vi "humidity_sensing_v_1.vi"() -> ()   [LabVIEW 2014]
doc: "This example shows how to configure a measurement and take a reading."
uses:
  <instrlib>/Keithley 24XX/Public/Data/Read (Single Point).vi
  <instrlib>/Keithley 24XX/Keithley 24XX.lvlib
panel:
  out "xxxxx":string
  in  "xxxxx":path=path "C:/Users/Administrator/Documents/Device-characterization-setup/IV-Trace/Data/dumb/2015_xx_xx_xxxx_xx_keithley_resistivity_001.txt"
  out "xxx":cluster{sgl[], i32[]}(graph)
  out "Data Real Time  Current":string
  in  "Data Real Time Current":path=path "C:/Users/Administrator/Documents/Device-characterization-setup/IV-Trace/Data/dumb/2015_xx_xx_xxxx_xx_keithley_resistivity_001.txt"
  out "Current-Sample Number":cluster{sgl[], i32[]}(graph)
  out "Analog Data 4":sgl(graph)
  out "Analog Data 3":sgl(graph)
  in  "loop num":dbl=1.0
  out "Data Resistivity":string
  in  "Data Resistivity":path=path "C:/Users/Administrator/Documents/Device-characterization-setup/IV-Trace/Data/dumb/2015_xx_xx_xxxx_xx_keithley_resistivity_001.txt"
  out "Resistance-Voltage":cluster{sgl[], sgl[]}(graph)
  in  "current multiplier":dbl=1.0
  out "Data IV Keithley":string
  in  "Data IV Keithley":path=path "C:/Users/Administrator/Documents/Device-characterization-setup/IV-Trace/Data/dumb/2015_xx_xx_xxxx_xx_keithley_001.txt"
  out "IV Curve":cluster{sgl[], dbl[]}(graph)
  in  "Stop Voltage/Current":dbl=2.0
  in  "Step":dbl=1.0
  in  "Source Mode  (0: Voltage)":u16(ring) items=["Voltage", "Current"]
  in  "Compliance  Level (0.1)":dbl=1.0
  in  "Start Voltage/Current":dbl
  in  "Enable Resistance Auto Range (T:Enable)":bool
  in  "Enable Current Auto Range (T:Enable)":bool=TRUE
  in  "Enable Voltage Auto Range (T:Enable)":bool
  in  "Resistance Manual Range (1.0)":dbl=1.0
  in  "Current Manual Range (1.0)":dbl=1.0
  in  "Voltage Manual Range (1.0)":dbl=1.0
  out "Resistance":sgl
  out "Current":sgl
  out "Voltage":sgl
  in  "Serial Configuration":T1={"Baud Rate"=9600, "Parity"=0, "Data Bits"=8, "Stop Bits"=10, "Flow Control"=0} {"Flow Control" items=["None", "XON/XOFF", "RTS/CTS", "XON/XOFF & RTS/CTS", "DTR/DSR", "XON/XOFF & DTR/DSR"]; "Stop Bits" items=["1.0"=10, "1.5"=15, "2.0"=20]; "Data Bits" items=["7"=7, "8"=8]; "Parity" items=["None", "Odd", "Even", "Mark", "Space"]; "Baud Rate" items=["300"=300, "600"=600, "1200"=1200, "2400"=2400, "4800"=4800, "9600"=9600, "19200"=19200]}
  in  "VISA resource name":refnum<visa-resource-name>="GPIB9::24::INSTR"
  # "NanoBEEs 2015-IV Tracer v1.0"
  # "Source Settings"
  # "GPIB9::24::INSTR"
  # "Voltage Range Settings"
  # "Current Range Settings"
  # "This multiplies the current value\nwith the number that entered, in order\nto  graph lower current values."
  # "Resistance Range Settings"
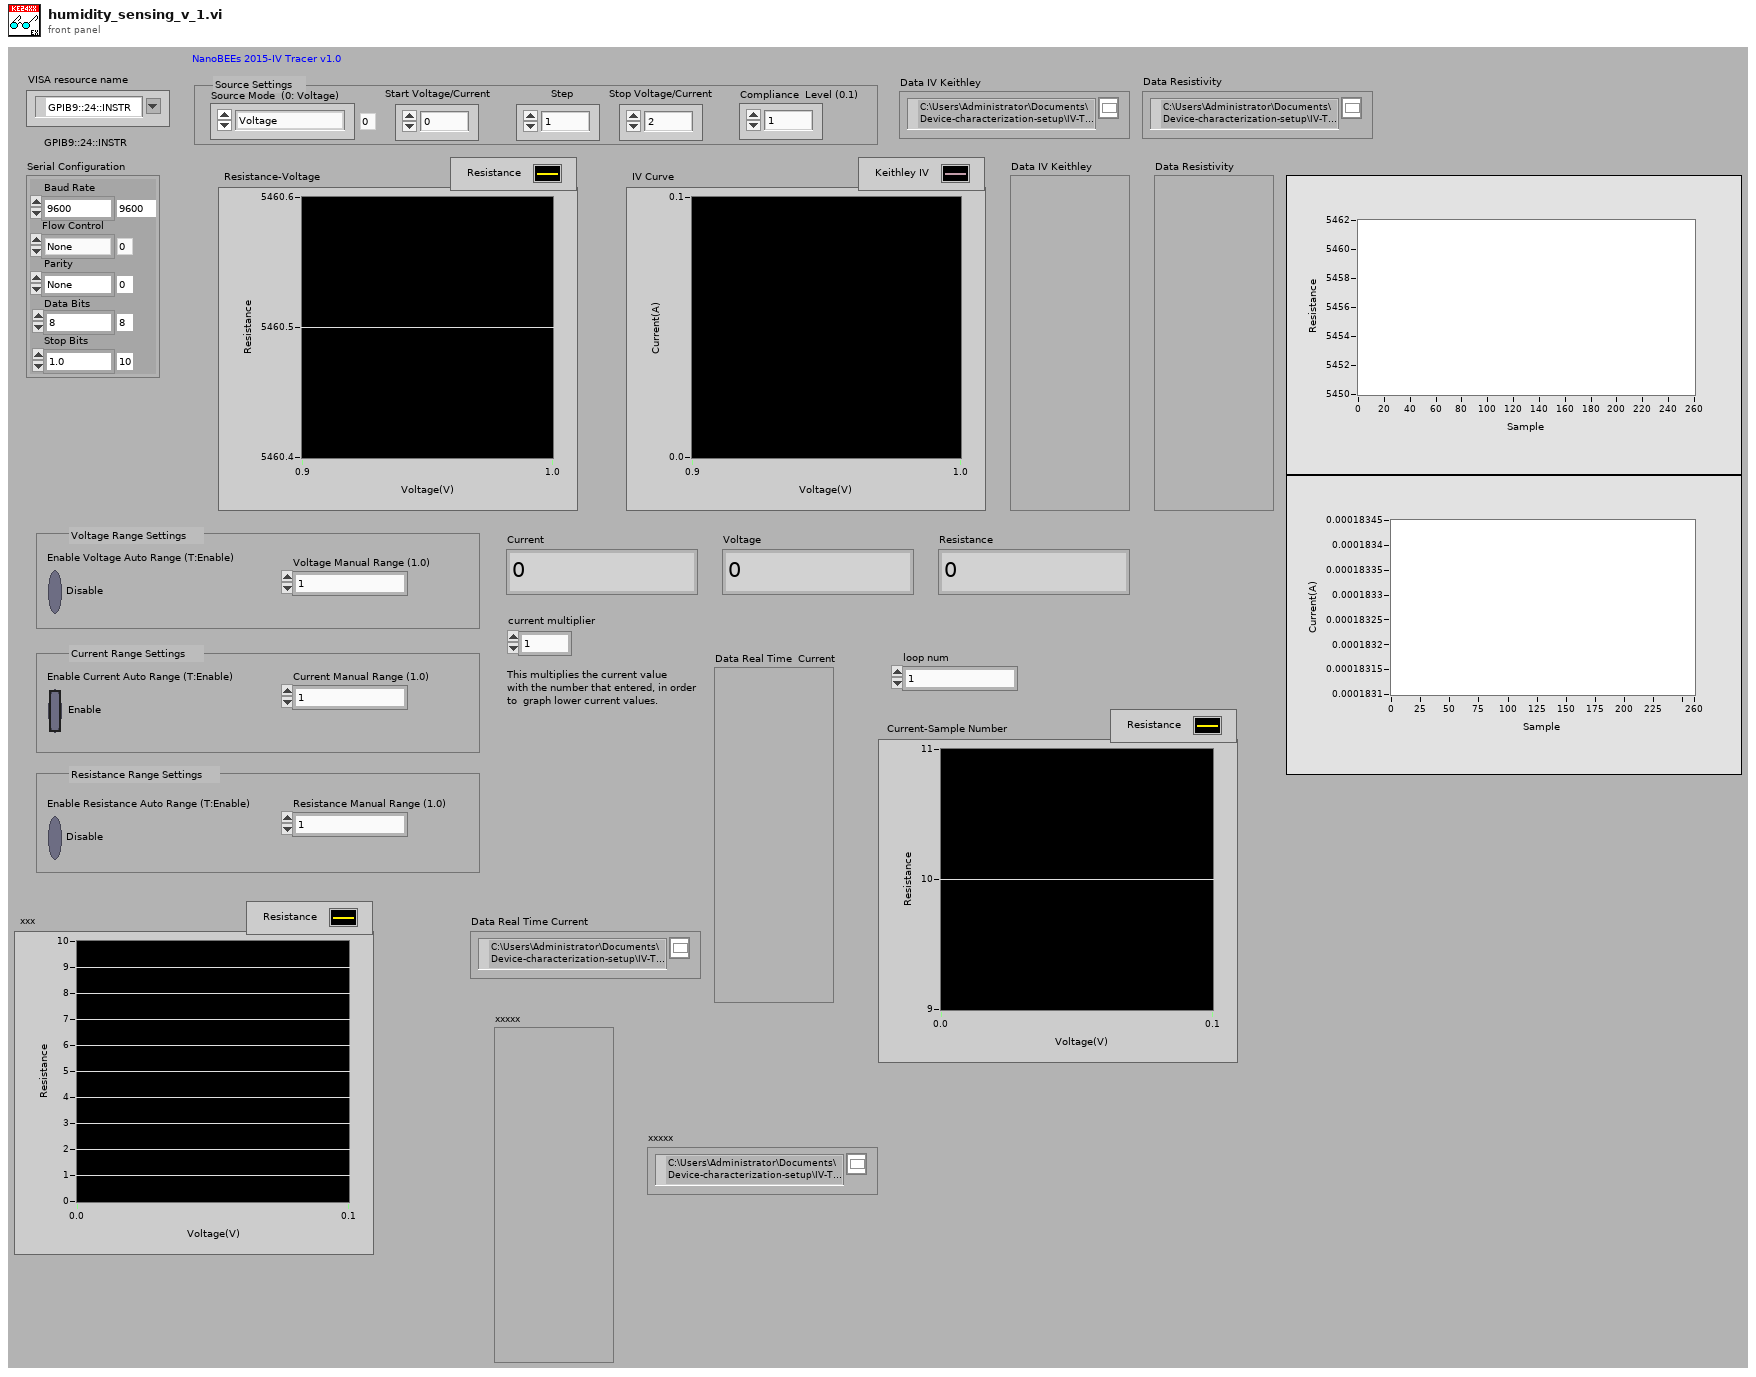
[diagram p1: front panel]
types:
  T1 = cluster{"Baud Rate":u32, "Parity":u16, "Data Bits":u16, "Stop Bits":u16, "Flow Control":u16}
  T2 = enum16{"open", "replace", "create", "open or create", "replace or create", "replace or create with confirmation"}
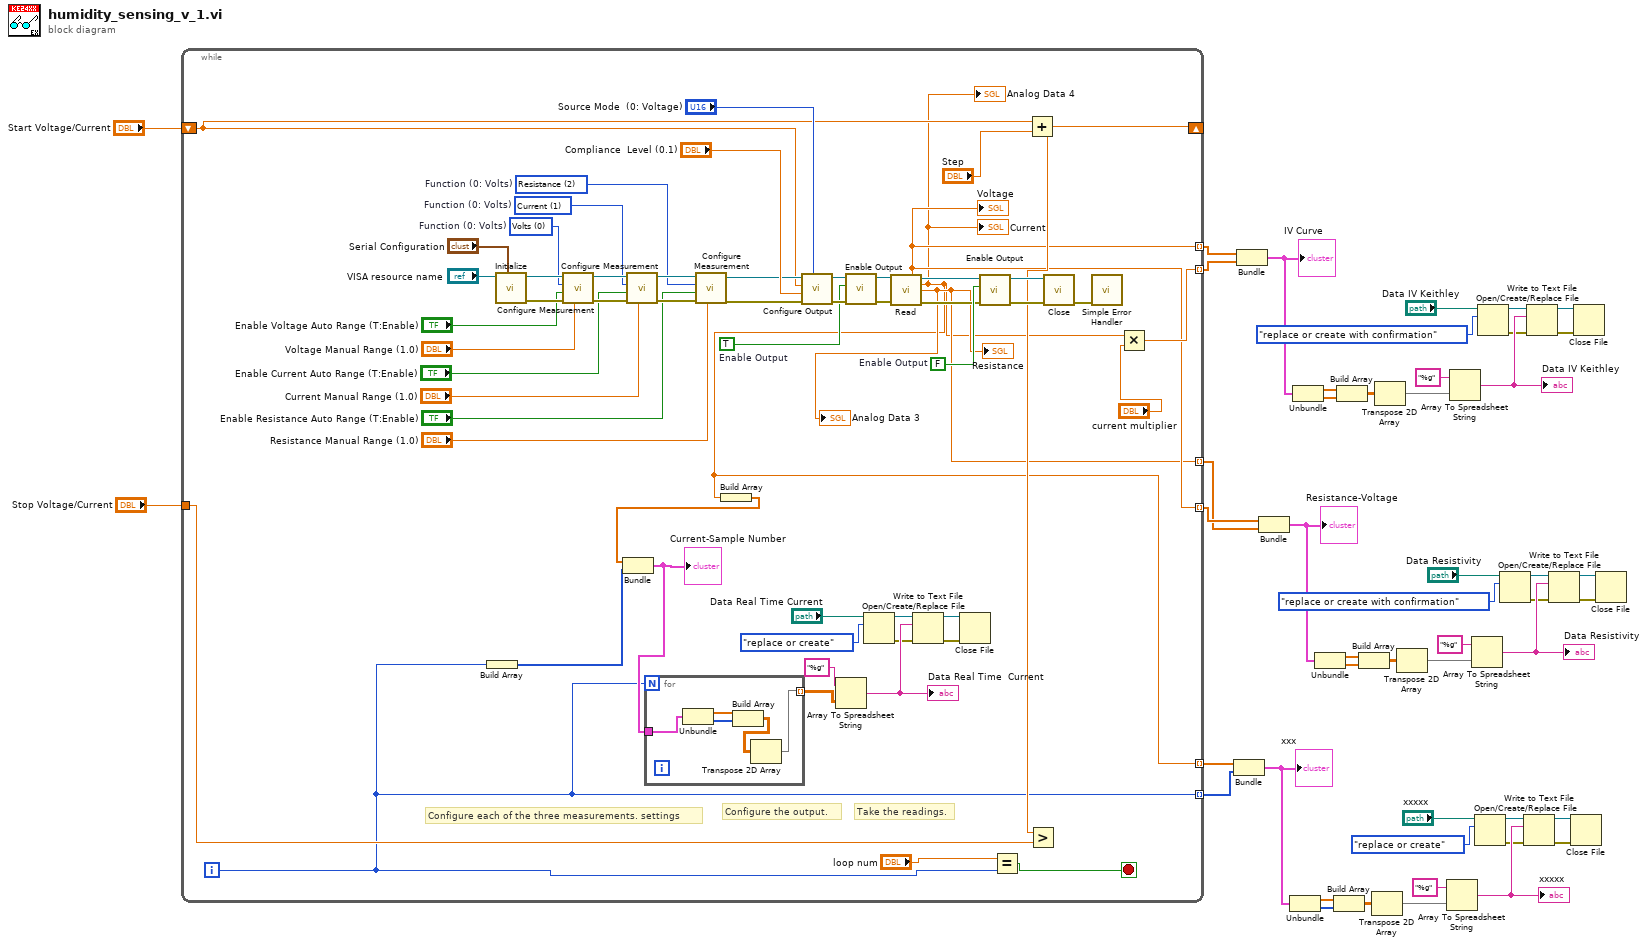
[diagram p0: block diagram]
diagram:
  n1 = while {
    shift-right: [w66] -> _
    shift-left: "Start Voltage/Current" -> [w71]
    tunnel: "Stop Voltage/Current" -> [w69]
    tunnel: [w68] -> w32 mode=indexing
    tunnel: [w65] -> w31 mode=indexing
    tunnel: [w51] -> w16 mode=indexing
    tunnel: [w65] -> w17 mode=indexing
    tunnel: [w49] -> w2 mode=indexing
    tunnel: [w48] -> w1 mode=indexing
    i -> [w48]
    stop <- w64 stop-if-true
    w75 = TRUE  # Enable Output
    w85 = FALSE  # Enable Output
    w92 = u16 2 items=["Volts", "Current", "Resistance"]  # Function (0: Volts)
    w93 = u16 1 items=["Volts", "Current", "Resistance"]  # Function (0: Volts)
    w94 = u16 0 items=["Volts", "Current", "Resistance"]  # Function (0: Volts)
    # "Take the readings."
    # "Configure the output."
    # "Configure each of the three measurements. settings"
    n2 = Build Array(w48) -> (w50:i32[])
    n3 = call <instrlib>:"Initialize.vi"("Serial Configuration"="Serial Configuration", "VISA resource name"="VISA resource name") -> ("error out"=w99:errorcluster, "VISA resource name out"=w100:refnum<visa-resource-name>)  [unwired: 8 in]
    n4 = call <instrlib>:"Configure Measurement.vi"("Manual Range (1.0)"="Voltage Manual Range (1.0)", "error in (no error)"=w99, "Enable Auto Range (T:Enable)"="Enable Voltage Auto Range (T:Enable)", "Function (0: Volts)"=w94, "VISA resource name"=w100) -> ("error out"=w97:errorcluster, "VISA resource name out"=w98:refnum<visa-resource-name>)  [unwired: 5 in]
    n5 = call <instrlib>:"Configure Measurement.vi"("Manual Range (1.0)"="Current Manual Range (1.0)", "error in (no error)"=w97, "Enable Auto Range (T:Enable)"="Enable Current Auto Range (T:Enable)", "Function (0: Volts)"=w93, "VISA resource name"=w98) -> ("error out"=w96:errorcluster, "VISA resource name out"=w95:refnum<visa-resource-name>)  [unwired: 5 in]
    n6 = call <instrlib>:"Configure Measurement.vi"("Manual Range (1.0)"="Resistance Manual Range (1.0)", "error in (no error)"=w96, "Enable Auto Range (T:Enable)"="Enable Resistance Auto Range (T:Enable)", "Function (0: Volts)"=w92, "VISA resource name"=w95) -> ("error out"=w74:errorcluster, "VISA resource name out"=w73:refnum<visa-resource-name>)  [unwired: 5 in]
    n7 = call <instrlib>:"Configure Output.vi"("Source Mode  (0: Voltage)"="Source Mode  (0: Voltage)", "error in (no error)"=w74, "Compliance  Level (0.1)"="Compliance  Level (0.1)", "Output Level (0)"=w71, "VISA resource name"=w73) -> ("error out"=w76:errorcluster, "VISA resource name out"=w77:refnum<visa-resource-name>)  [unwired: 5 in]
    n8 = call <instrlib>:"Enable Output.vi"("error in (no error)"=w76, "Enable Output (T: Enable)"=w75, "VISA resource name"=w77) -> ("error out"=w79:errorcluster, "VISA resource name out"=w78:refnum<visa-resource-name>)  [unwired: 7 in]
    n9 = Open/Create/Replace File(file path (use dialog)="Data Real Time Current", operation (0:open)=T2."replace or create") -> (refnum out=w62:refnum<file>, error out=w57:errorcluster)  [unwired: 4 in, 1 out]
    n10 = call-poly <instrlib>:"Read.vi"("VISA resource name"=w78, "error in (no error)"=w79) -> ("Voltage"=w65:sgl, "VISA resource name out"=w80:refnum<visa-resource-name>, "Current"=w49:sgl, "Resistance"=w51:sgl, "error out"=w81:errorcluster)  [unwired: 7 in, 2 out]
    "Voltage" <- w65
    "Current" <- w49
    "Resistance" <- w51
    "Analog Data 3" <- w51
    "Analog Data 4" <- w49
    n11 = Build Array(w49) -> (w55:sgl[])
    n12 = Bundle(w55, w50) -> (w54:cluster{sgl[], i32[]})  [unwired: 1 out]
    "Current-Sample Number" <- w54
    n13 = for {
      N: w48 -> [_]
      tunnel: w54 -> [w108]
      tunnel: [w104] -> w53 mode=indexing
      n14 = Unbundle(w108) -> (w107:sgl[], w106:i32[])
      n15 = Build Array(w107, w106) -> (w105:sgl[][])
      n16 = Transpose 2D Array(2D array=w105) -> (transposed array=w104:sgl[][])
    }
    n17 = Array To Spreadsheet String(array=w53, 3:"%g" ("format string")) -> (spreadsheet string=w63:string)  [unwired: 1 in]
    "Data Real Time  Current" <- w63
    n18 = Write to Text File(file (use dialog)=w62, text=w63, error in=w57) -> (refnum out=w59:refnum<file>, error out=w58:errorcluster)  [unwired: 2 out]
    n19 = Close File(refnum=w59, error in=w58) -> ()  [unwired: 2 out]
    n20 = call <instrlib>:"Enable Output.vi"("error in (no error)"=w81, "Enable Output (T: Enable)"=w85, "VISA resource name"=w80) -> ("error out"=w82:errorcluster, "VISA resource name out"=w83:refnum<visa-resource-name>)  [unwired: 7 in]
    n21 = Equal?(x="loop num", y=w48) -> (x = y?=w64:bool)
    n22 = Add(x=w71, y="Step") -> (x+y=w66:dbl)
    n23 = Greater?(x=w66, y=w69) -> ()  [unwired: 1 out]
    n24 = call <instrlib>:"Close.vi"("error in (no error)"=w82, "VISA resource name"=w83) -> ("error out"=w103:errorcluster)  [unwired: 9 in]
    n25 = call <vilib>:"Simple Error Handler.vi"("error in (no error)"=w103) -> ()  [unwired: 4 in, 5 out]
    n26 = Multiply(x=w49, y="current multiplier") -> (x*y=w68:dbl)
  }
  n27 = Bundle(w2, w1) -> (w9:cluster{sgl[], i32[]})  [unwired: 1 out]
  "xxx" <- w9
  n28 = Bundle(w31, w32) -> (w39:cluster{sgl[], dbl[]})  [unwired: 1 out]
  "IV Curve" <- w39
  n29 = Bundle(w17, w16) -> (w24:cluster{sgl[], sgl[]})  [unwired: 1 out]
  "Resistance-Voltage" <- w24
  n30 = Unbundle(w9) -> (w10:sgl[], w11:i32[])
  n31 = Unbundle(w39) -> (w40:sgl[], w41:dbl[])
  n32 = Unbundle(w24) -> (w25:sgl[], w26:sgl[])
  n33 = Build Array(w10, w11) -> (w12:sgl[][])
  n34 = Build Array(w40, w41) -> (w42:dbl[][])
  n35 = Build Array(w25, w26) -> (w27:sgl[][])
  n36 = Transpose 2D Array(2D array=w12) -> (transposed array=w14:sgl[][])
  n37 = Transpose 2D Array(2D array=w42) -> (transposed array=w44:dbl[][])
  n38 = Transpose 2D Array(2D array=w27) -> (transposed array=w29:sgl[][])
  n39 = Array To Spreadsheet String(array=w14, 3:"%g" ("format string")) -> (spreadsheet string=w15:string)  [unwired: 1 in]
  "xxxxx" <- w15
  n40 = Array To Spreadsheet String(array=w44, 3:"%g" ("format string")) -> (spreadsheet string=w45:string)  [unwired: 1 in]
  "Data IV Keithley" <- w45
  n41 = Array To Spreadsheet String(array=w29, 3:"%g" ("format string")) -> (spreadsheet string=w30:string)  [unwired: 1 in]
  "Data Resistivity" <- w30
  n42 = Open/Create/Replace File(file path (use dialog)="xxxxx", operation (0:open)=T2."replace or create") -> (refnum out=w8:refnum<file>, error out=w3:errorcluster)  [unwired: 4 in, 1 out]
  n43 = Open/Create/Replace File(file path (use dialog)="Data IV Keithley", operation (0:open)=T2."replace or create with confirmation") -> (refnum out=w38:refnum<file>, error out=w33:errorcluster)  [unwired: 4 in, 1 out]
  n44 = Open/Create/Replace File(file path (use dialog)="Data Resistivity", operation (0:open)=T2."replace or create with confirmation") -> (refnum out=w23:refnum<file>, error out=w18:errorcluster)  [unwired: 4 in, 1 out]
  n45 = Write to Text File(file (use dialog)=w8, text=w15, error in=w3) -> (refnum out=w5:refnum<file>, error out=w4:errorcluster)  [unwired: 2 out]
  n46 = Write to Text File(file (use dialog)=w38, text=w45, error in=w33) -> (refnum out=w35:refnum<file>, error out=w34:errorcluster)  [unwired: 2 out]
  n47 = Write to Text File(file (use dialog)=w23, text=w30, error in=w18) -> (refnum out=w20:refnum<file>, error out=w19:errorcluster)  [unwired: 2 out]
  n48 = Close File(refnum=w5, error in=w4) -> ()  [unwired: 2 out]
  n49 = Close File(refnum=w35, error in=w34) -> ()  [unwired: 2 out]
  n50 = Close File(refnum=w20, error in=w19) -> ()  [unwired: 2 out]
